vi "呱呱叫.vi"(8 "error in (no error)":errorcluster caption="错误输入（无错误）", 11 "鸭子 输入":refnum<class "鸭子.lvclass">) -> (0 "error out":errorcluster caption="错误输出", 3 "鸭子 输出":refnum<class "鸭子.lvclass">)   [LabVIEW 2018, in "鸭子库.lvlib" / "鸭子.lvclass"]
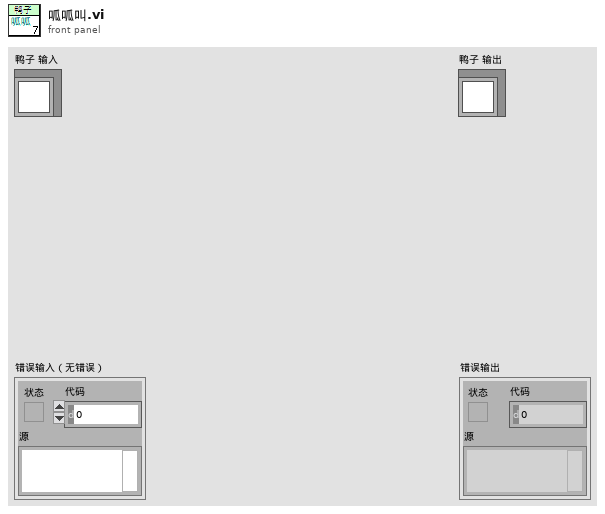
[diagram p1: front panel]
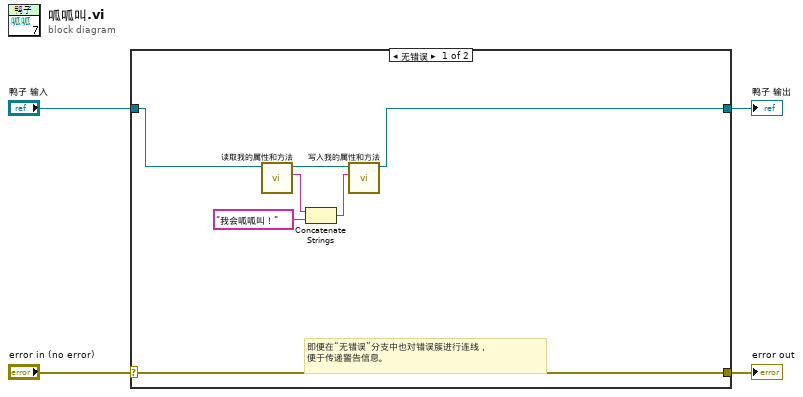
[diagram p0: block diagram]
diagram:
  n1 = case shown="无错误" "error in (no error)" {
    selector: "error in (no error)" -> [w11 w13]
    tunnel: [w11 w13] -> w3
    tunnel: [w6 w12] -> w1
    tunnel: "鸭子 输入" -> [w8 w12]
    frame No Error {
      # "即便在“无错误”分支中也对错误簇进行连线，\n便于传递警告信息。"
      n2 = call "读取我的属性和方法.vi"("鸭子输入"=w8) -> ("我的属性和方法"=w10:string, "鸭子输出"=w7:refnum<class "鸭子.lvclass">)  [unwired: 8 in, 1 out]
      n3 = Concatenate Strings(w10, "我会呱呱叫！" ("字符串")) -> (w5:string)
      n4 = call "写入我的属性和方法.vi"("我的属性和方法"=w5, "鸭子输入"=w7) -> ("鸭子输出"=w6:refnum<class "鸭子.lvclass">)  [unwired: 8 in, 1 out]
    }
    frame Error {
    }
  }
  "error out" <- w3
  "鸭子 输出" <- w1
